vi "VNA_Easy_Data.vi"(4 "stop/span":dbl=10000000000.0 format="%.2e", 5 "start/center":dbl=1000000000.0 format="%.2e", 6 "sweep time (sec)":dbl=0.1 format="%.2f", 7 "sweep type (0 : linear)":u16(ring) items=["linear sweep", "logarithmic sweep", "frequency list", "CW time sweep", "power sweep"], 8 "error in (no error)":errorcluster, 9 "num points":u16(ring)=5 items=["3", "11", "21 ('20) / 26 ('53)", "51", "101", "201", "401", "801", "1601"], 10 "measurement (0 : S11)":u16(ring) items=["Ref1 : Forward S11 (A/R)", "Trans: Forward S21 (B/R)", "Trans: Reverse S12 (A/R)", "Ref1: Reverse S22 (B/R)", "Analog In, AUX input", "A/R", "B/R", "A/B", "A", "B", "R"], 11 "VISA Refnum in":refnum<visa-resource-name>) -> (0 "error out":errorcluster, 2 "Data":cluster{dbl[], sgl[]}, 3 "VISA Refnum out":refnum<visa-resource-name>)   [LabVIEW 2019]
uses:
  <instrlib>/Agilent 87XX Series/Agilent 87XX Series.lvlib
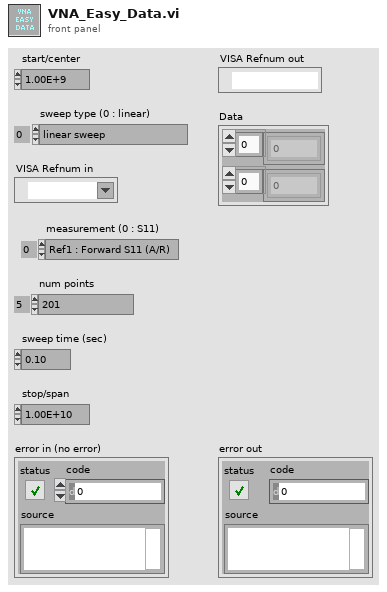
[diagram p1: front panel]
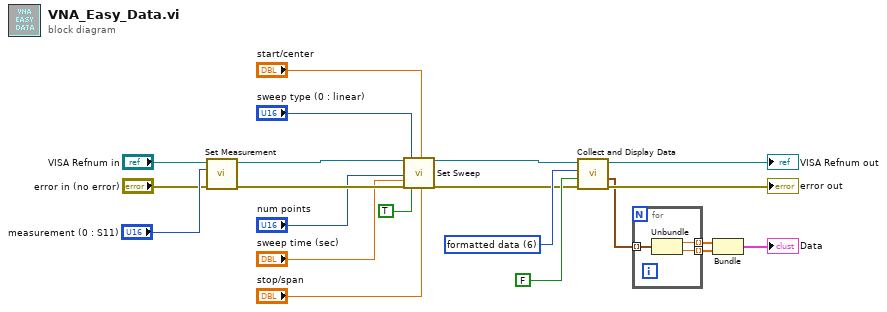
[diagram p0: block diagram]
diagram:
  w12 = u16 6 items=["raw data array 1", "raw data array 2", "raw data array 3", "raw data array 4", "error-corrected data", "error-corrected trace memory", "formatted data", "formatted memory", "formatted data / memory", "formatted data - memory"] ("data type (6 : formatted data)")
  n1 = call <instrlib>:"Set Measurement.vi"("error in (no error)"="error in (no error)", "measurement (0 : S11)"="measurement (0 : S11)", "VISA resource name"="VISA Refnum in") -> ("error out"=w16:errorcluster, "VISA resource name out"=w14:refnum<visa-resource-name>)  [unwired: 7 in]
  n2 = call <instrlib>:"Set Sweep.vi"("VISA resource name"=w14, "num points"="num points", "sweep time (sec)"="sweep time (sec)", "error in (no error)"=w16, "sweep type (0 : linear)"="sweep type (0 : linear)", "t: start/stop  f: center/span"=TRUE, "start/center"="start/center", "stop/span"="stop/span") -> ("VISA resource name out"=w2:refnum<visa-resource-name>, "error out"=w1:errorcluster)  [unwired: 10 in]
  n3 = call <instrlib>:"Collect and Display Data.vi"("error in (no error)"=w1, "save to file"=FALSE, "data type (6 : formatted data)"=w12, "VISA resource name"=w2) -> ("error out"=→"error out":errorcluster, "data values"=w9:cluster{"real / stim":dbl, "imag / resp":sgl}[], "VISA resource name out"=→"VISA Refnum out":refnum<visa-resource-name>)  [unwired: 4 in, 1 out]
  n4 = for {
    tunnel: w9 -> [w24] mode=indexing
    tunnel: [w23] -> w10 mode=indexing
    tunnel: [w22] -> w11 mode=indexing
    n5 = Unbundle(w24) -> ("real / stim"=w23:dbl, "imag / resp"=w22:sgl)
  }
  n6 = Bundle(w10, w11) -> (→"Data":cluster{dbl[], sgl[]})  [unwired: 1 in]
